vi "LIA 4SOS.vi"(6 "lock-in.iir config0 0":T2={"b0"=0.015777587890625, "b1"=-0.030517578125, "-a1"=1.9578399658203125, "-a2"=-0.9589080810546875}, 7 "lock-in.iir enable0 0":bool, 9 "input valid":bool, 10 "lock-in.iir decimation0 0":fxp<+,4,4> format="%#_3g", 11 "IQ_Data_In":T1) -> (1 "output valid":bool, 3 "IQ_Data_Out":T1)   [LabVIEW 2018]
uses:
  Shared/SOS/Controls/IIR_Coeffs.ctl
  <instrlib>/_niInstr/DSP/v1/Shared/Public/IQ Data.ctl
  <instrlib>/_niInstr/DSP/v1/Shared/niInstr DSP v1 Shared.lvlib
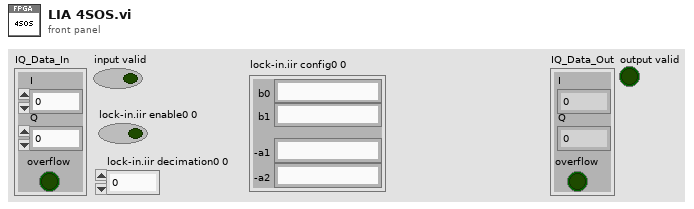
[diagram p1: front panel]
types:
  T1 = typedef "niInstr DSP v1 Shared.lvlib/IQ Data.ctl" = cluster{"I":fxp<+/-,18,1>, "Q":fxp<+/-,18,1>, "overflow":bool}
  T2 = typedef "IIR_Coeffs.ctl" = cluster{"b0":fxp<+/-,18,2>, "b1":fxp<+/-,18,2>, "-a1":fxp<+/-,18,2>, "-a2":fxp<+/-,18,2>}
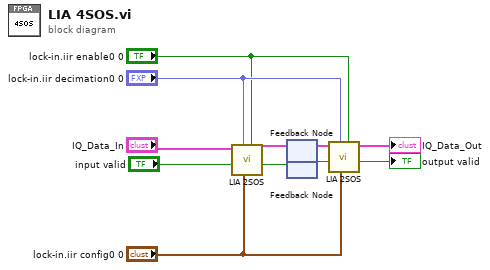
[diagram p0: block diagram]
diagram:
  n1 = call "LIA 2SOS.vi"("lock-in.iir enable0 0"="lock-in.iir enable0 0", "lock-in.iir config0 0"="lock-in.iir config0 0", "lock-in.iir decimation0 0"="lock-in.iir decimation0 0", "input valid"="input valid", "IQ_Data_In"="IQ_Data_In") -> ("output valid"=w8:bool, "IQ_Data_Out"=w11:T1)  [unwired: 5 in]
  n2 = feedback-in #1(w11) -> ()
  n3 = feedback #1() -> (w7:T1)  [unwired: 1 in]
  n4 = feedback-in #2(w8) -> ()
  n5 = feedback #2() -> (w2:bool)  [unwired: 1 in]
  n6 = call "LIA 2SOS.vi"("lock-in.iir enable0 0"="lock-in.iir enable0 0", "lock-in.iir config0 0"="lock-in.iir config0 0", "lock-in.iir decimation0 0"="lock-in.iir decimation0 0", "input valid"=w2, "IQ_Data_In"=w7) -> ("output valid"=→"output valid":bool, "IQ_Data_Out"=→"IQ_Data_Out":T1)  [unwired: 5 in]
